vi "Fetch.vi"   [LabVIEW 2020, in "Keithley DMM6500 DAQ6500 Series.lvlib"]
doc: "Retrieve data from instrument."
uses:
  <instrlib>/Keithley DMM6500 DAQ6500 Series/Keithley DMM6500 DAQ6500 Series.lvlib
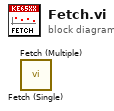
[diagram p0: block diagram]
diagram:
  n1 = call <instrlib>:"Fetch (Single).vi"() -> ()  [unwired: 9 in, 3 out]
  n2 = call <instrlib>:"Fetch (Multiple).vi"() -> ()  [unwired: 9 in, 3 out]
